vi "motortestMeng4XY.vi"() -> ()   [LabVIEW 2014]
doc: "Shows how to perform a relative motor move."
uses:
  <vilib>/Utility/inputDevices.llb/joystickAcquire.vi
  <vilib>/Utility/inputDevices.llb/closeJoystick.vi
panel:
  out "Position Z":sgl
  out "Position X":sgl=7.9123425
  in  "Stop":bool
  in  "MG17Motor Z":refnum<k7>(container)
  in  "Motor settings (Z)":cluster{"Vmax (mm/s)":sgl, "Acc (mm/s/s)":sgl}={"Vmax (mm/s)"=0.03, "Acc (mm/s/s)"=1.0}
  out "Position Y":sgl=4.4431553
  in  "Motor settings (X,Y)":cluster{"Vmax (mm/s)":sgl, "Acc (mm/s/s)":sgl}={"Vmax (mm/s)"=0.1, "Acc (mm/s/s)"=1.0}
  in  "Motor Limits":T1={"XMAX"=8.5, "XMIN"=5.0, "YMAX"=6.0, "YMIN"=4.0, "ZMAX"=0.1, "ZMIN"=-0.3}
  in  "MG17Motor Y":refnum<k7>(container)
  out "axis info":T2={"X axis"=-256, "Y axis"=-256, "Z axis"=32767, "X axis rotation"=0, "Y axis rotation"=0, "Z axis rotation"=0, "U axis"=0, "V axis"=0}
  out "button info":T3
  in  "MG17Motor X":refnum<k7>(container)
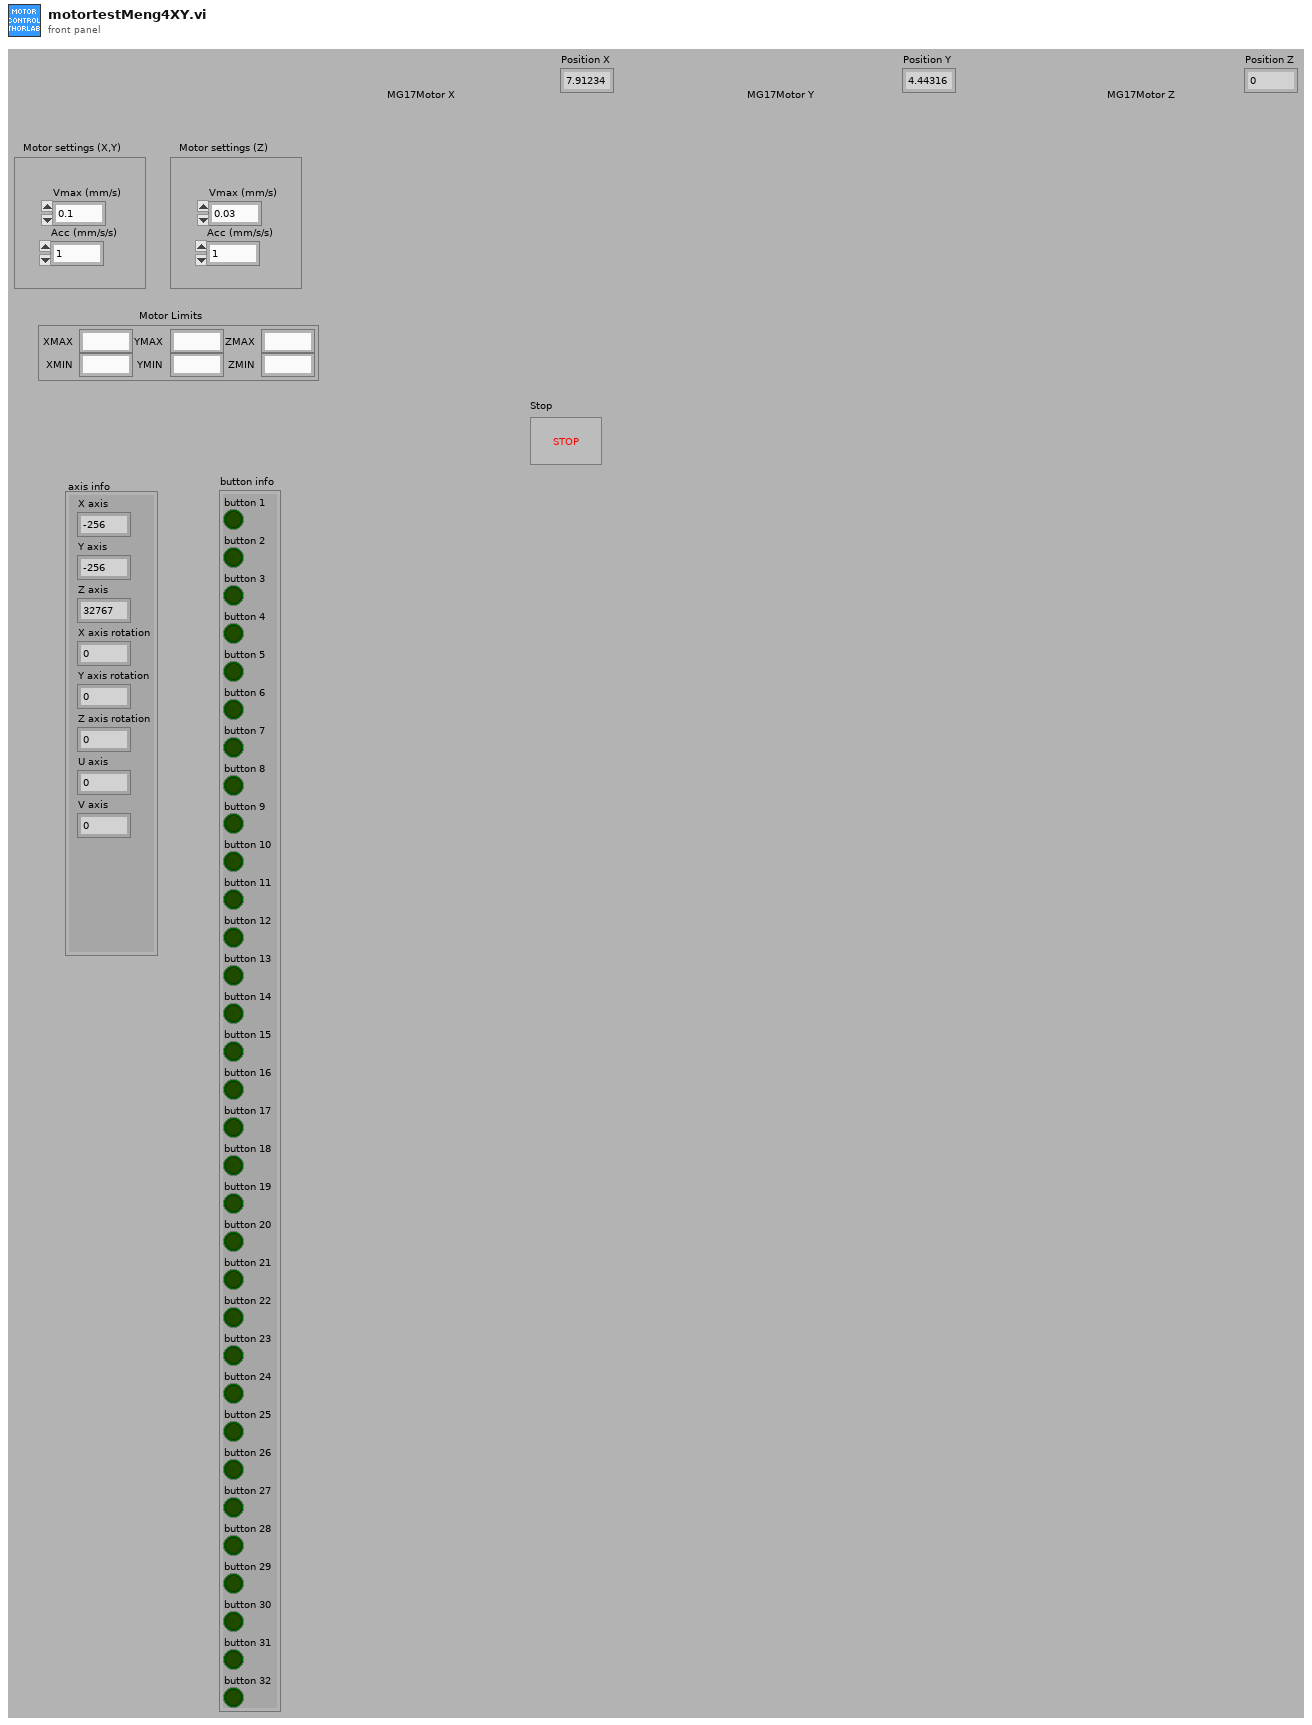
[diagram p1: front panel]
types:
  T1 = cluster{"XMAX":sgl, "XMIN":sgl, "YMAX":sgl, "YMIN":sgl, "ZMAX":sgl, "ZMIN":sgl}
  T2 = cluster{"X axis":i32, "Y axis":i32, "Z axis":i32, "X axis rotation":i32, "Y axis rotation":i32, "Z axis rotation":i32, "U axis":i32, "V axis":i32}
  T3 = cluster{"button 1":bool, "button 2":bool, "button 3":bool, "button 4":bool, "button 5":bool, "button 6":bool, "button 7":bool, "button 8":bool, "button 9":bool, "button 10":bool, "button 11":bool, "button 12":bool, "button 13":bool, "button 14":bool, "button 15":bool, "button 16":bool, "button 17":bool, "button 18":bool, "button 19":bool, "button 20":bool, "button 21":bool, "button 22":bool, "button 23":bool, "button 24":bool, "button 25":bool, "button 26":bool, "button 27":bool, "button 28":bool, "button 29":bool, "button 30":bool, "button 31":bool, "button 32":bool}
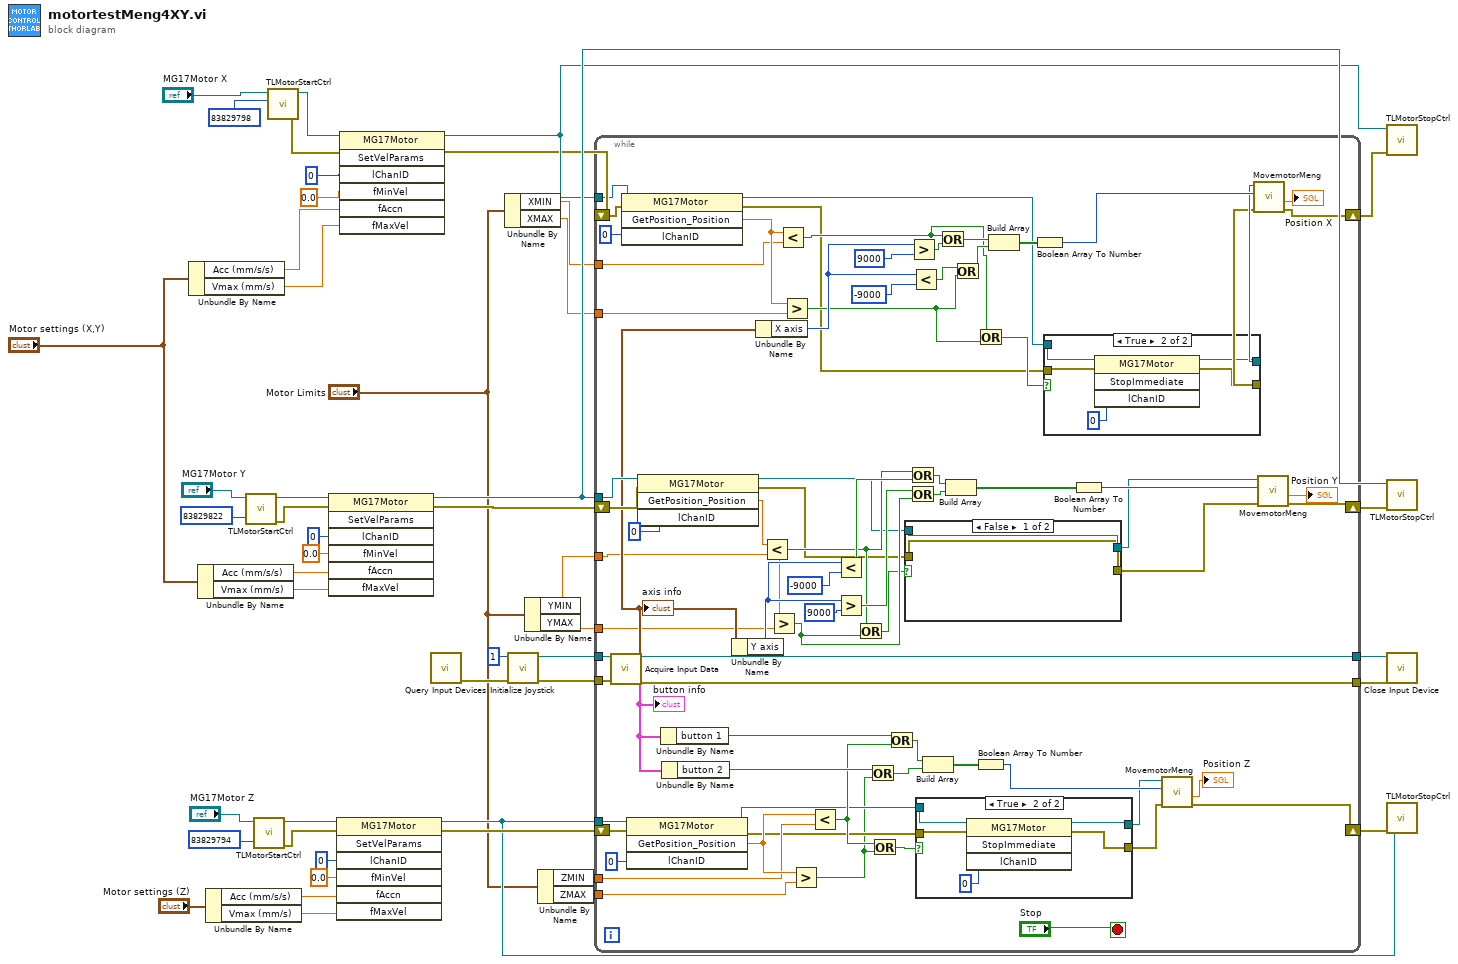
[diagram p0: block diagram]
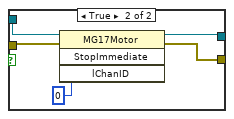
[diagram p2: hidden frame]
diagram:
  n1 = Unbundle By Name("Motor settings (X,Y)") -> ("Acc (mm/s/s)"=w32:sgl, "Vmax (mm/s)"=w31:sgl)
  n2 = Unbundle By Name("Motor settings (X,Y)") -> ("Acc (mm/s/s)"=w28:sgl, "Vmax (mm/s)"=w27:sgl)
  n3 = Unbundle By Name("Motor settings (Z)") -> ("Acc (mm/s/s)"=w16:sgl, "Vmax (mm/s)"=w17:sgl)
  n4 = call "TLMotorStartCtrl.vi"("SerialNum"=83829822 ("lChanID"), "Motor Ref"="MG17Motor Y") -> ("Error Out"=w29:errorcluster, "Motor Ref"=w30:refnum<k7>)  [unwired: 4 in]
  n5 = call "TLMotorStartCtrl.vi"("SerialNum"=83829794 ("lChanID"), "Motor Ref"="MG17Motor Z") -> ("Error Out"=w15:errorcluster, "Motor Ref"=w14:refnum<k7>)  [unwired: 4 in]
  n6 = call "TLMotorStartCtrl.vi"("SerialNum"=83829798 ("lChanID"), "Motor Ref"="MG17Motor X") -> ("Error Out"=w35:errorcluster, "Motor Ref"=w36:refnum<k7>)  [unwired: 4 in]
  n7 = invoke class="MG17Motor" method="SetVelParams"(reference=w30, error in=w29, "lChanID"=0, "fMinVel"=sgl 0.0, "fAccn"=w28, "fMaxVel"=w27) -> (reference out=w24:refnum<k7>, error out=w21:errorcluster)  [unwired: 1 in, 5 out]
  n8 = invoke class="MG17Motor" method="SetVelParams"(reference=w14, error in=w15, "lChanID"=0, "fMinVel"=sgl 0.0, "fAccn"=w16, "fMaxVel"=w17) -> (reference out=w8:refnum<k7>, error out=w10:errorcluster)  [unwired: 1 in, 5 out]
  n9 = invoke class="MG17Motor" method="SetVelParams"(reference=w36, error in=w35, "lChanID"=0, "fMinVel"=sgl 0.0, "fAccn"=w32, "fMaxVel"=w31) -> (reference out=w23:refnum<k7>, error out=w22:errorcluster)  [unwired: 1 in, 5 out]
  n10 = call <vilib>:"Query Input Devices.vi"() -> ("error out"=w47:errorcluster)  [unwired: 8 in, 3 out]
  n11 = Unbundle By Name("Motor Limits") -> ("XMIN"=w20:sgl, "XMAX"=w3:sgl)
  n12 = call <vilib>:"Initialize Joystick.vi"("error in (no error)"=w47, "device index"=1) -> ("error out"=w45:errorcluster, "device ID"=w46:refnum<k1>)  [unwired: 8 in]
  n13 = Unbundle By Name("Motor Limits") -> ("YMIN"=w5:sgl, "YMAX"=w4:sgl)
  n14 = Unbundle By Name("Motor Limits") -> ("ZMIN"=w7:sgl, "ZMAX"=w2:sgl)
  n15 = while {
    shift-left: w22 -> [w113]
    shift-right: [w106] -> w38
    tunnel: w23 -> [w108]
    tunnel: w46 -> [w124]
    tunnel: w45 -> [w123]
    tunnel: [w122] -> w44
    tunnel: [w121] -> w43
    tunnel: w24 -> [w89]
    shift-right: [w115] -> w37
    shift-left: w21 -> [w88]
    tunnel: w3 -> [w96]
    tunnel: w20 -> [w93]
    tunnel: w8 -> [w102]
    shift-right: [w103] -> w9
    shift-left: w10 -> [w101]
    tunnel: w7 -> [w75]
    tunnel: w4 -> [w84]
    tunnel: w5 -> [w81]
    tunnel: w2 -> [w63]
    stop <- "Stop" stop-if-true
    n16 = call-poly <vilib>:"Acquire Input Data.vi"("device ID"=w124, "error in (no error)"=w123) -> ("device ID 2"=w122:refnum<k1>, "axis info"=w86:T2, "button info"=w120:T3, "error out"=w121:errorcluster)  [unwired: 13 in, 1 out]
    "axis info" <- w86
    "button info" <- w120
    n17 = invoke class="MG17Motor" method="GetPosition_Position"(reference=w108, error in=w113, "lChanID"=0) -> (reference out=w58:refnum<k7>, error out=w59:errorcluster, "GetPosition_Position"=w94:sgl)  [unwired: 1 in, 1 out]
    n18 = invoke class="MG17Motor" method="GetPosition_Position"(reference=w102, error in=w101, "lChanID"=0) -> (reference out=w72:refnum<k7>, error out=w71:errorcluster, "GetPosition_Position"=w76:sgl)  [unwired: 1 in, 1 out]
    n19 = invoke class="MG17Motor" method="GetPosition_Position"(reference=w89, error in=w88, "lChanID"=0) -> (reference out=w50:refnum<k7>, error out=w52:errorcluster, "GetPosition_Position"=w82:sgl)  [unwired: 1 in, 1 out]
    n20 = Unbundle By Name(w120) -> ("button 1"=w98:bool)
    n21 = Unbundle By Name(w120) -> ("button 2"=w97:bool)
    n22 = Unbundle By Name(w86) -> ("Y axis"=w87:i32)
    n23 = Unbundle By Name(w86) -> ("X axis"=w109:i32)
    n24 = Less?(x=w82, y=w81) -> (x < y?=w55:bool)
    n25 = Greater?(x=w82, y=w84) -> (0:w54:bool)
    n26 = Less?(x=w94, y=w93) -> (x < y?=w61:bool)
    n27 = Greater?(x=w94, y=w96) -> (0:w62:bool)
    n28 = Greater?(x=w76, y=w63) -> (0:w68:bool)
    n29 = Less?(x=w76, y=w75) -> (x < y?=w74:bool)
    n30 = Less?(x=w87, y=-9000) -> (x < y?=w80:bool)
    n31 = Greater?(x=w87, y=9000) -> (0:w78:bool)
    n32 = Or(x=w55, y=w54) -> (x .or. y?=w53:bool)
    n33 = Or(x=w97, y=w68) -> (x .or. y?=w66:bool)
    n34 = Or(x=w74, y=w68) -> (x .or. y?=w73:bool)
    n35 = Or(x=w98, y=w74) -> (x .or. y?=w67:bool)
    n36 = case shown="False" w53 {
      tunnel: w50 -> [w126 w131]
      tunnel: w52 -> [w125 w130]
      tunnel: [w125 w129] -> w51
      tunnel: [w126 w128] -> w49
      frame False {
      }
      frame True {
        n37 = invoke class="MG17Motor" method="StopImmediate"(reference=w131, error in=w130, "lChanID"=0) -> (reference out=w128:refnum<k7>, error out=w129:errorcluster)  [unwired: 1 in, 2 out]
      }
    }
    n38 = Or(x=w55, y=w80) -> (x .or. y?=w79:bool)
    n39 = Or(x=w78, y=w54) -> (x .or. y?=w83:bool)
    n40 = Greater?(x=w109, y=9000) -> (0:w92:bool)
    n41 = Less?(x=w109, y=-9000) -> (x < y?=w95:bool)
    n42 = case shown="True" w73 {
      tunnel: w72 -> [w140 w145]
      tunnel: w71 -> [w139 w144]
      tunnel: [w139 w143] -> w70
      tunnel: [w140 w142] -> w69
      frame False {
      }
      frame True {
        n43 = invoke class="MG17Motor" method="StopImmediate"(reference=w145, error in=w144, "lChanID"=0) -> (reference out=w142:refnum<k7>, error out=w143:errorcluster)  [unwired: 1 in, 2 out]
      }
    }
    n44 = Build Array(w67, w66) -> (w105:bool[])
    n45 = Or(x=w61, y=w92) -> (x .or. y?=w91:bool)
    n46 = Build Array(w79, w83) -> (w119:bool[])
    n47 = Or(x=w95, y=w62) -> (x .or. y?=w90:bool)
    n48 = Or(x=w61, y=w62) -> (x .or. y?=w60:bool)
    n49 = Boolean Array To Number(Boolean array=w105) -> (number=w104:u32)
    n50 = Build Array(w91, w90) -> (w110:bool[])
    n51 = Boolean Array To Number(Boolean array=w110) -> (number=w107:u32)
    n52 = case shown="True" w60 {
      tunnel: w58 -> [w133 w138]
      tunnel: w59 -> [w132 w137]
      tunnel: [w132 w136] -> w56
      tunnel: [w133 w135] -> w57
      frame False {
      }
      frame True {
        n53 = invoke class="MG17Motor" method="StopImmediate"(reference=w138, error in=w137, "lChanID"=0) -> (reference out=w135:refnum<k7>, error out=w136:errorcluster)  [unwired: 1 in, 2 out]
      }
    }
    n54 = Boolean Array To Number(Boolean array=w119) -> (number=w116:u32)
    n55 = call "MovemotorMeng.vi"("error in (no error)"=w70, "Numeric"=w104, "Automation Refnum in"=w69) -> ("error out"=w103:errorcluster, "Position"=→"Position Z":sgl)  [unwired: 6 in, 1 out]
    n56 = call "MovemotorMeng.vi"("error in (no error)"=w56, "Numeric"=w107, "Automation Refnum in"=w57) -> ("error out"=w106:errorcluster, "Position"=→"Position X":sgl)  [unwired: 6 in, 1 out]
    n57 = call "MovemotorMeng.vi"("error in (no error)"=w51, "Numeric"=w116, "Automation Refnum in"=w49) -> ("error out"=w115:errorcluster, "Position"=→"Position Y":sgl)  [unwired: 6 in, 1 out]
  }
  n58 = call "TLMotorStopCtrl.vi"("Error In (No Error)"=w38, "Motor Ref"=w23) -> ()  [unwired: 4 in, 2 out]
  n59 = call "TLMotorStopCtrl.vi"("Error In (No Error)"=w37, "Motor Ref"=w24) -> ()  [unwired: 4 in, 2 out]
  n60 = call-poly <vilib>:"Close Input Device.vi"("error in (no error)"=w43, "device ID"=w44) -> ()  [unwired: 8 in, 1 out]
  n61 = call "TLMotorStopCtrl.vi"("Error In (No Error)"=w9, "Motor Ref"=w8) -> ()  [unwired: 4 in, 2 out]
